vi "Close_old.vi"(8 "error in (no error)":errorcluster, 11 "Vaisala in":refnum<class "Vaisala.lvclass">) -> (0 "error out":errorcluster, 3 "Vaisala out":refnum<class "Vaisala.lvclass">)   [LabVIEW 2014, in "Vaisala.lvclass"]
uses:
  Vaisala.lvclass
  Reusable/Session APIs/Text Communication/Text Device Session.lvclass
  Vaisala.lvclass/Vaisala.ctl
  <userlib>/_Session Fwk/Session - Root.lvclass
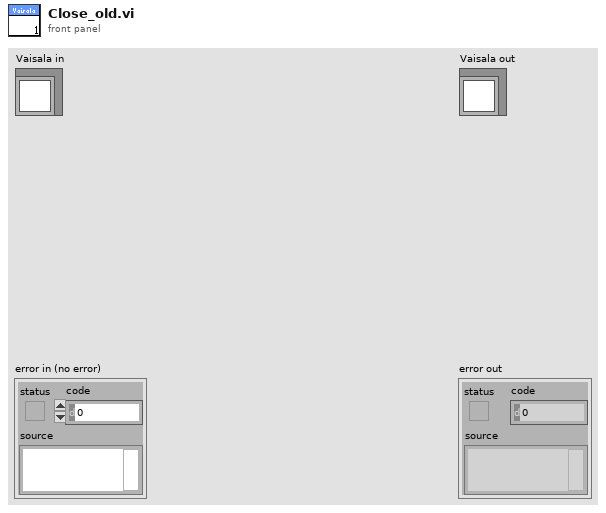
[diagram p1: front panel]
types:
  T1 = typedef "Session - Root.lvclass/Session Handle.ctl" = refnum<data-value>
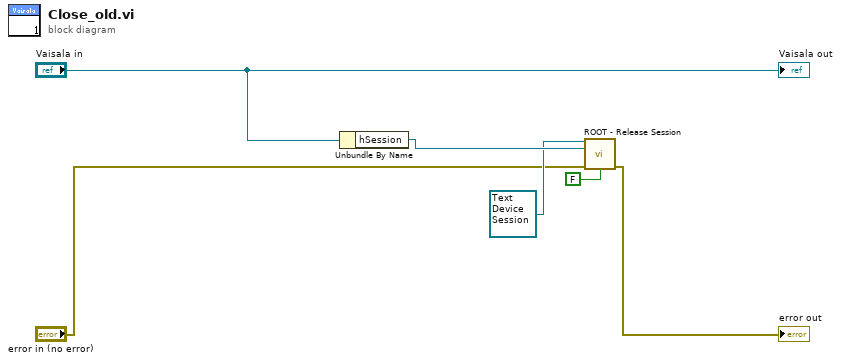
[diagram p0: block diagram]
diagram:
  n1 = Unbundle By Name("Vaisala in") -> ("hSession"=w5:T1)
  n2 = call <userlib>:"ROOT - Release Session.vi"("OBJ - Session in"=refnum<class "Text Device Session.lvclass"> refnum ("Text Session"), "Session Handle in"=w5, "error in (no error)"="error in (no error)", "force destroy? (F)"=FALSE) -> ("error out"=→"error out":errorcluster)  [unwired: 9 in, 2 out]
  "Vaisala out" <- "Vaisala in"
